vi "Izhikevich_primitive_v005.vi"(0 "UDP Network Connection in":refnum<k16>, 1 "b":dbl, 2 "a":dbl, 3 "I":dbl, 5 "c":dbl, 7 "d":dbl, 9 "v(t)":dbl, 11 "error in (no error)":errorcluster, 12 "u(t)":dbl, 13 "Numeric":dbl, 14 "Address selector":i32[](array[numeric])) -> (4 "UDP Network Connection out":refnum<k16>, 6 "v(t+dt)":dbl, 8 "u(t+dt)":dbl, 15 "error out":errorcluster)   [LabVIEW 2021]
panel:
  in  "time":dbl
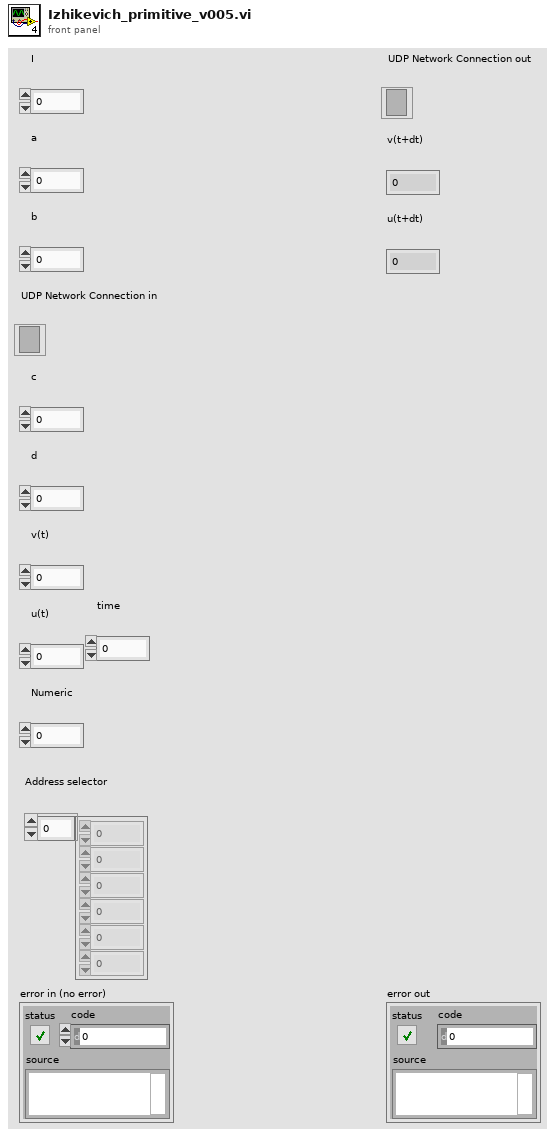
[diagram p1: front panel]
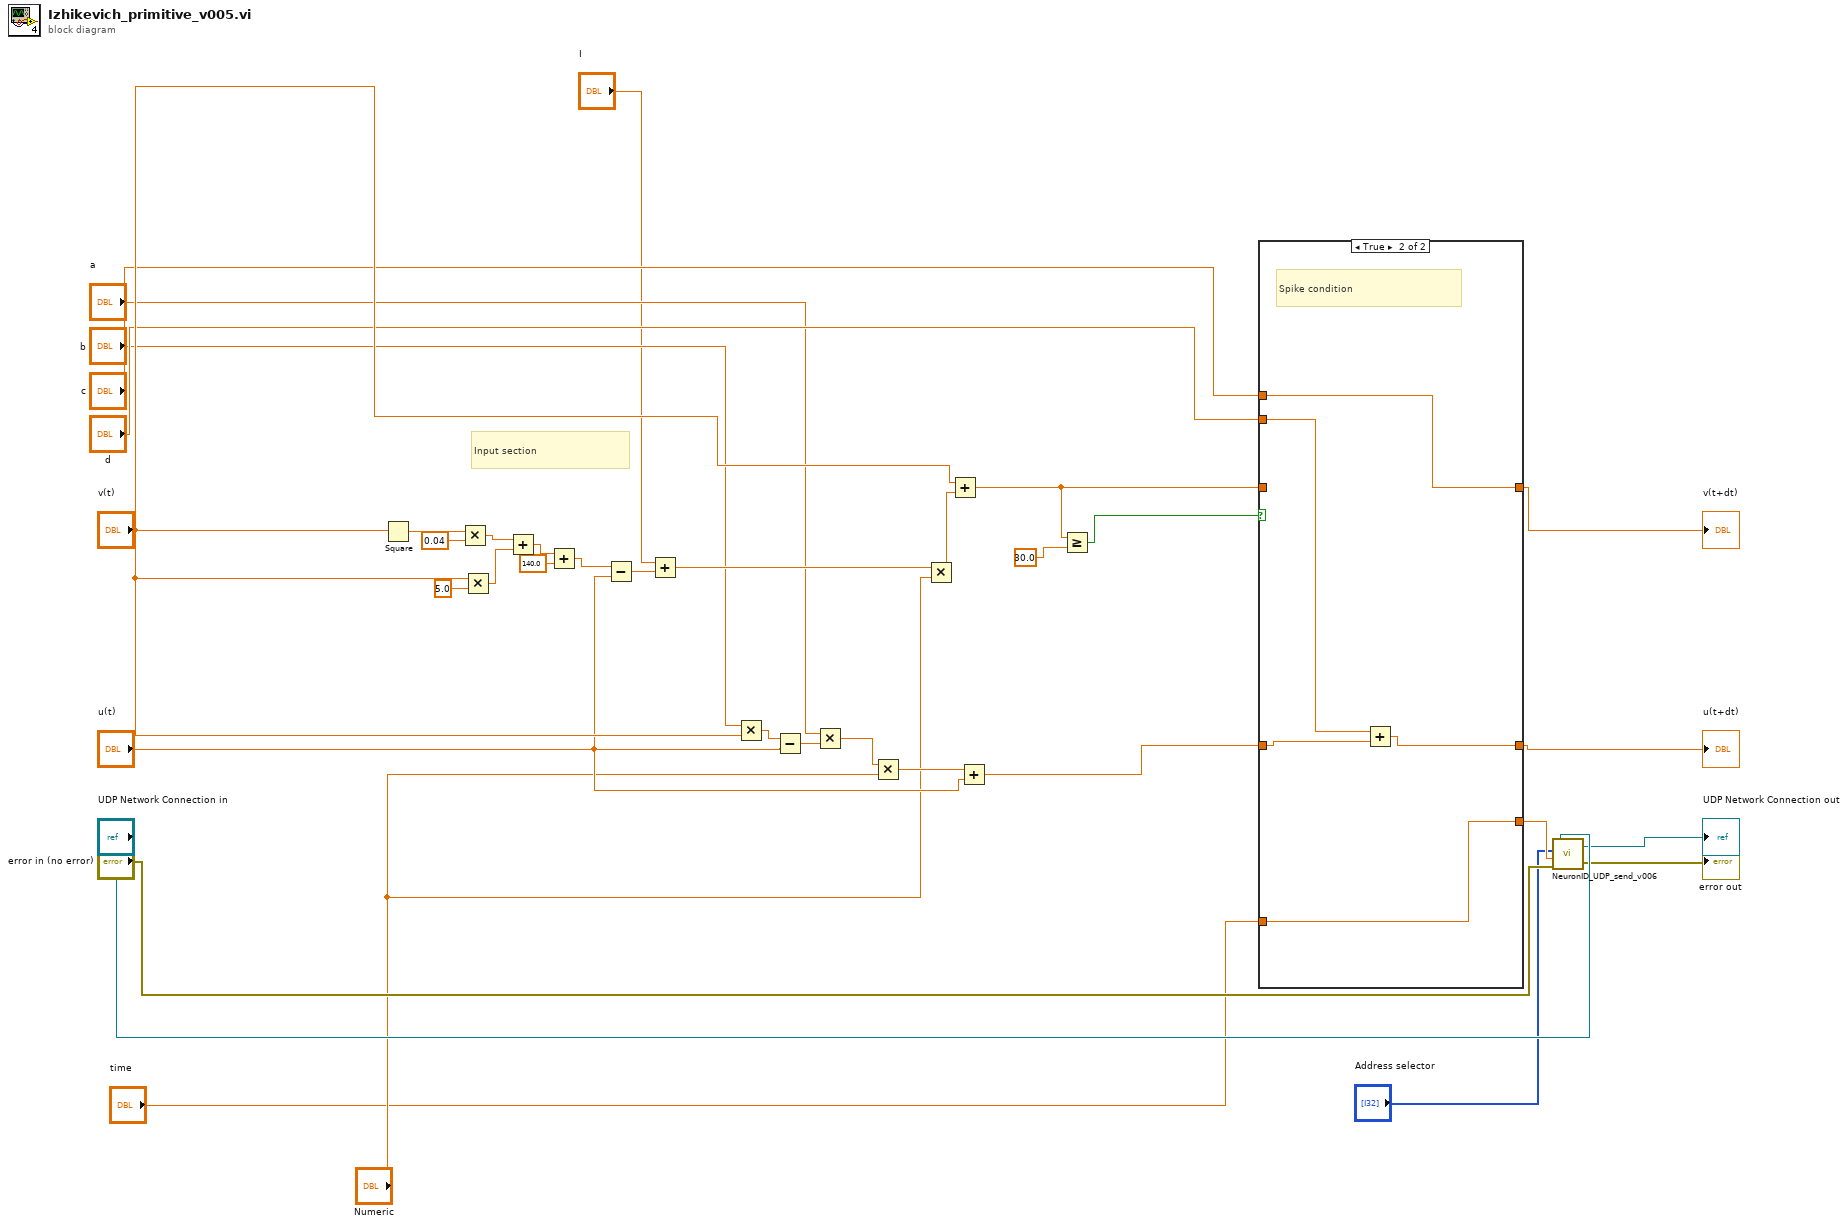
[diagram p0: block diagram]
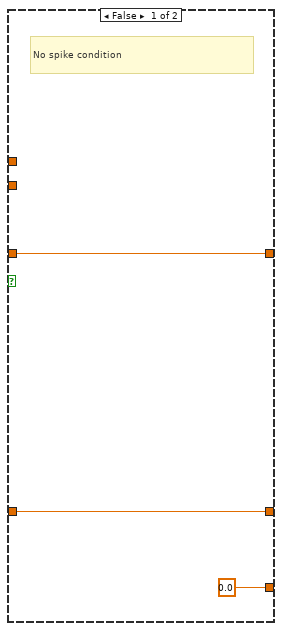
[diagram p2: hidden frame]
diagram:
  # "Input section"
  n1 = Square(x="v(t)") -> (x^2=w6:dbl)
  n2 = Multiply(x=w6, y=0.04) -> (x*y=w8:dbl)
  n3 = Multiply(x="v(t)", y=5.0) -> (x*y=w10:dbl)
  n4 = Add(x=w8, y=w10) -> (x+y=w11:dbl)
  n5 = Add(x=w11, y=140.0) -> (x+y=w13:dbl)
  n6 = Subtract(x=w13, y="u(t)") -> (x-y=w14:dbl)
  n7 = Add(x="I", y=w14) -> (x+y=w21:dbl)
  n8 = Multiply(x="b", y="v(t)") -> (x*y=w17:dbl)
  n9 = Subtract(x=w17, y="u(t)") -> (x-y=w18:dbl)
  n10 = Multiply(x="a", y=w18) -> (x*y=w20:dbl)
  n11 = Multiply(x=w20, y="Numeric") -> (x*y=w24:dbl)
  n12 = Multiply(x=w21, y="Numeric") -> (x*y=w23:dbl)
  n13 = Add(x="v(t)", y=w23) -> (x+y=w33:dbl)
  n14 = Add(x=w24, y="u(t)") -> (x+y=w26:dbl)
  n15 = Greater Or Equal?(x=w33, y=30.0) -> (x >= y?=w34:bool)
  n16 = case shown="True" w34 {
    tunnel: [w39 w41] -> w25
    tunnel: w26 -> [w39 w43]
    tunnel: w33 -> [w38 _]
    tunnel: [w38 w44] -> w27
    tunnel: "c" -> [_ w44]
    tunnel: "d" -> [_ w42]
    tunnel: [0.0 ("Neuron ID") w40] -> w5
    tunnel: "time" -> [_ w40]
    frame False {
      # "No spike condition"
    }
    frame True {
      # "Spike condition"
      n17 = Add(x=w42, y=w43) -> (x+y=w41:dbl)
    }
  }
  "v(t+dt)" <- w27
  "u(t+dt)" <- w25
  n18 = call "NeuronID_UDP_send_v006.vi"("error in (no error)"="error in (no error)", "Neuron ID"=w5, "Address selector"="Address selector", "UDP Network Connection in"="UDP Network Connection in") -> ("error out"=→"error out":errorcluster, "UDP Network Connection out"=→"UDP Network Connection out":refnum<k16>)
